vi "Get.vi"(8 "error in (no error)":errorcluster, 11 "Ref":refnum<queue>) -> (0 "error out":errorcluster, 2 "Variant":variant, 3 "Ref out":refnum<queue>)   [LabVIEW 2016, in "SEQ.lvlib"]
doc: "Get the Single Element Queued (SEQ) based variable in variant format."
uses:
  SEQ.lvlib
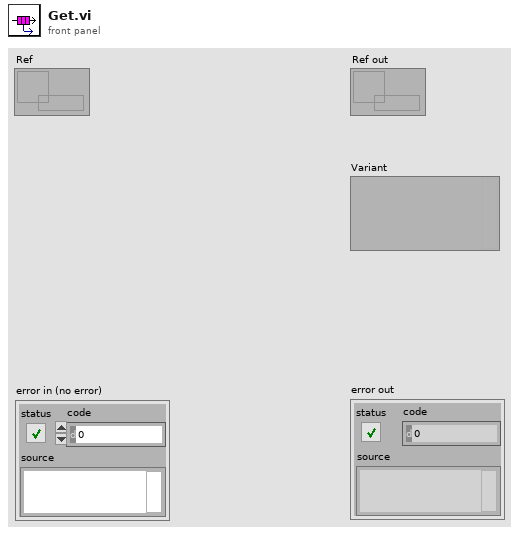
[diagram p1: front panel]
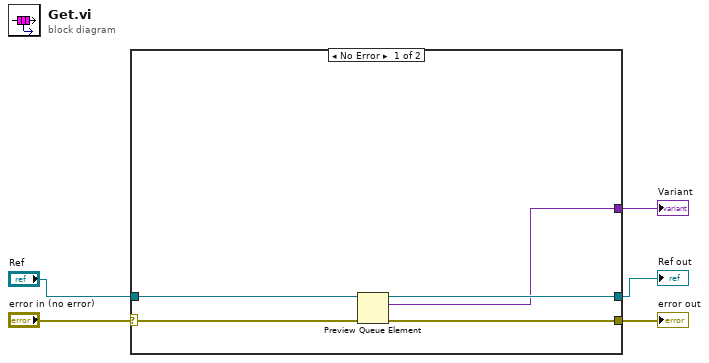
[diagram p0: block diagram]
diagram:
  n1 = case shown="No Error" "error in (no error)" {
    selector: "error in (no error)" -> [w10 w12]
    tunnel: [w6 w12] -> w5
    tunnel: "Ref" -> [w9 w11]
    tunnel: [w8 w11] -> w1
    tunnel: [w7 _] -> w3
    frame No Error {
      n2 = Preview Queue Element(queue=w9, error in (no error)=w10) -> (queue out=w8:refnum<queue>, element=w7:variant, error out=w6:errorcluster)  [unwired: 1 in, 1 out]
    }
    frame Error {
    }
  }
  "error out" <- w5
  "Variant" <- w3
  "Ref out" <- w1
